vi "Distance to RPM_V1.vi"(3 "Personality":string, 4 "Target Distance":dbl) -> (1 "Shooter RPM Control":dbl)   [LabVIEW 2013]
panel:
  in  "Sting Offset":dbl(knob)=5.025737873391023 scale=-100.0..100.0
  in  "Sister-Sting Offset":dbl(knob)=6.675453710228453 scale=-100.0..200.0
  # "Started at -20"
  # "Started at 180"
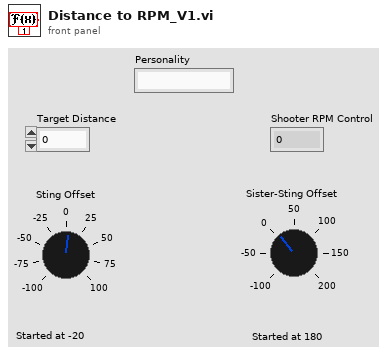
[diagram p1: front panel]
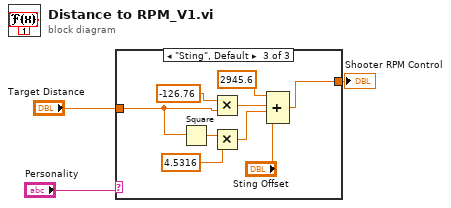
[diagram p0: block diagram]
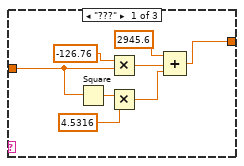
[diagram p2: hidden frame]
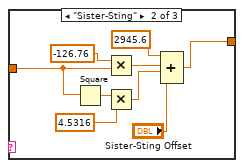
[diagram p3: hidden frame]
diagram:
  n1 = case shown="\"Sting\", Default" "Personality" {
    tunnel: [w5 w14 w26] -> w2
    tunnel: "Target Distance" -> [w4 w13 w22]
    frame "???" {
      n2 = Square(x=w4) -> (x^2=w6:dbl)
      n3 = Multiply(x=-126.76, y=w4) -> (x*y=w9:dbl)
      n4 = Multiply(x=w6, y=4.5316) -> (x*y=w10:dbl)
      n5 = Compound Arithmetic op=ADD(2945.6 ("value"), w9, w10) -> (w5:dbl)
    }
    frame "Sister-Sting" {
      n6 = Square(x=w13) -> (x^2=w20:dbl)
      n7 = Multiply(x=-126.76, y=w13) -> (x*y=w17:dbl)
      n8 = Multiply(x=w20, y=4.5316) -> (x*y=w16:dbl)
      n9 = Compound Arithmetic op=ADD(2945.6 ("value"), w17, w16, "Sister-Sting Offset") -> (w14:dbl)
    }
    frame "Sting", Default {
      n10 = Square(x=w22) -> (x^2=w29:dbl)
      n11 = Multiply(x=-126.76, y=w22) -> (x*y=w25:dbl)
      n12 = Multiply(x=w29, y=4.5316) -> (x*y=w24:dbl)
      n13 = Compound Arithmetic op=ADD(2945.6 ("value"), w25, w24, "Sting Offset") -> (w26:dbl)
    }
  }
  "Shooter RPM Control" <- w2
